vi "CheckFreeSpot.vi"(8 "ErrorIn":errorcluster, 9 "MinError":i32, 10 "MaxError":i32, 11 "ConnectionIn":refnum<class "Connection.lvclass">) -> (0 "ErrorOut":errorcluster, 1 "Valid":bool, 2 "ErrorCode":i32, 3 "ConnectionOut":refnum<class "Connection.lvclass">, 4 "Existing":bool)   [LabVIEW 2021, in "ErrorDefinitionSQLite.lvclass"]
uses:
  ErrorDefinitionSQLite.lvclass
  <vilib>/drjdpowell/SQLite Library/SQL Connection/Connection.lvclass
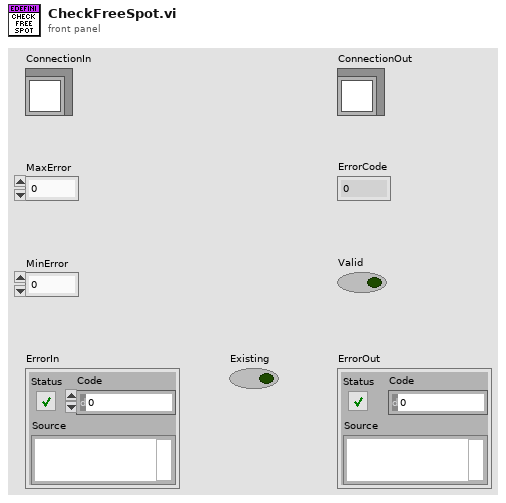
[diagram p1: front panel]
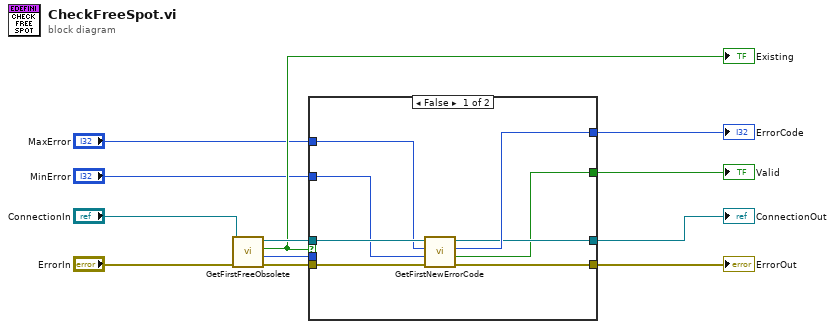
[diagram p0: block diagram]
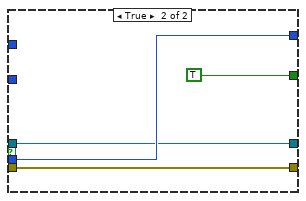
[diagram p2: hidden frame]
diagram:
  n1 = call "GetFirstFreeObsolete.vi"("ErrorIn"="ErrorIn", "ConnectionIn"="ConnectionIn") -> ("ErrorOut"=w11:errorcluster, "FirstFreeObsolete"=w4:i32, "Valid"=w3:bool, "ConnectionOut"=w8:refnum<class "Connection.lvclass">)  [unwired: 6 in]
  "Existing" <- w3
  n2 = case shown="False" w3 {
    tunnel: w8 -> [w18 w21]
    tunnel: w11 -> [w20 w24]
    tunnel: [w17 w23] -> w7
    tunnel: [w16 w21] -> w6
    tunnel: [w19 w24] -> w10
    tunnel: [w15 TRUE ("Valid")] -> w5
    tunnel: w4 -> [_ w23]
    tunnel: "MinError" -> [w14 _]
    tunnel: "MaxError" -> [w13 _]
    frame False {
      n3 = call "GetFirstNewErrorCode.vi"("ErrorIn"=w20, "MinError"=w14, "MaxError"=w13, "ConnectionIn"=w18) -> ("ErrorOut"=w19:errorcluster, "Valid"=w15:bool, "NewErrorCode"=w17:i32, "ConnectionOut"=w16:refnum<class "Connection.lvclass">)  [unwired: 4 in]
    }
    frame True {
    }
  }
  "ErrorCode" <- w7
  "Valid" <- w5
  "ConnectionOut" <- w6
  "ErrorOut" <- w10
